vi "Motor_Plus_Impedance_controller_using_force_feedback_only.vi"() -> ()   [LabVIEW 2016]
uses:
  <vilib>/Platform/TimedLoop/XDataNode/timing_clust.ctl
  <vilib>/Platform/TimedLoop/XDataNode/nitl_modes.ctl
  <vilib>/Platform/TimedLoop/XDataNode/wakeup.ctl
  <vilib>/Platform/TimedLoop/XDataNode/loadnilvce.vi
  <vilib>/Motion/Express/_s/nimc.fb.resetPosition.resetPosition.axis.vi
  <vilib>/Motion/Express/_s/nimc.fb.read.readFaults.axis.vi
  <vilib>/Motion/Express/_s/nimc.fb.read.readExecutionStatus.axis.vi
  <vilib>/Motion/Express/_s/nimc.fb.straightLineMove.startStraightLineMove.axis.modeRelative.0.vi
  <vilib>/Motion/Express/_s/nimc.fb.read.readExecutionData.axis.vi
  <vilib>/Motion/Express/_s/nimc.fb.straightLineMove.startStraightLineMove.axis.modeAbsolute.0.vi
  <vilib>/Motion/Express/_s/nimc.ax.power.power.axis.vi
  <vilib>/Motion/Express/_s/nimc.fb.stopMove.stop.axis.modeDecelerate.vi
  <vilib>/Motion/Express/_s/nimc.ex.power.power.axis.vi
  <vilib>/Platform/TimedLoop/XDataNode/XDataNode.xnode
  <vilib>/Motion/BlockNode/FB.NIMotion.xnode
  <vilib>/functionblocks/FB Property/FB Overlay DBL.ctl
  <vilib>/Platform/TimedLoop/XDataNode/XDNodeRunTimeDep.lvlib
panel:
  in  "Tab Control":enum32{"Record", "PID Check", "Load Cell Check"}(tab)
  out "Crank Position, rev":dbl(knob) scale=-100.0..100.0
  out "Crank Speed, rev/s":dbl(knob) scale=0.0..300.0
  out "Motor Torque, Nm":dbl(knob) scale=-5.0..5.0
  out "Load Cell Force, N":dbl(knob) scale=-50.0..50.0
  out "Recording?":bool
  in  "Record Data?":bool
  in  "Path":path=path "C:/ni-rt/LabVIEW Data/Ashley Carter"
  in  "File Name:":string="2015_03_31_60rpm_20rev_B_1.tdms"
  in  "Prime New File?":bool
  out "File being written to:":path
  out "FIFO Timer, Sec":dbl
  out "FIFO motor position, rev":dbl
  out "FIFO motor velocity, rev/s":dbl
  out "FIFO motor torque, Nm":dbl
  out "FIFO Load cell, V":dbl
  out "FIFO File logging trigger":dbl
  out "# FIFO elements remaining in buffer":u32
  out "Data File Crank Angle Sample Resolution, degrees of crank rotation":dbl
  out "Motor Control PID Check":cluster{dbl, dbl}(graph)
  out "Load Cell Check":cluster{dbl, dbl, dbl}(graph)
  out "Logging loop duration, ms":u32
  out "Control loop duration, ms":u32
  out "RPM LIMITING!":bool
  in  "desired motor\nposition":dbl
  in  "Move to Position?":bool
  in  "Reset Position?":bool
  out "fault occurred":bool
  out "System reported fault codes":i32[](array[numeric])
  out "Load cell, V":dbl format="%.3f"
  out "motor torque, Nm":dbl format="%.3f"
  out "motor velocity, rev/s":dbl format="%.3f"
  out "motor position, rev":dbl format="%.3f"
  out "Timer, sec":dbl format="%.3f"
  out "drive enabled":bool
  out "axis enabled":bool
  out "move complete":bool
  in  "STOP VI":bool
  in  "Enable Axis Control":bool
  in  "Enable Motor Drive":bool
  in  "crank rpm":dbl=60.0
  in  "crank no. revolutions":dbl=5.0
  in  "EMERGENCY MOTOR STOP":bool
  in  "Start Test?":bool
  # "Impedance Motor Controller"
  # "Impedance Control Basic Data Recording and PID Tuning"
  # "(This only stops the move, the drive remains enabled!!!)"
  # "Crank RPM and no. Revolutions"
  # "Raw Data from System"
  # "Suggested process to align above reported motor position to test rig TDC:\n\nWith the Enable Motor Drive and Enable Axis Control switches set to off\nmanually rotate the 'engine' to BDC then click Enable Motor Control and \nEnable Axis Control. 'motor position, rev' above then reports a value. Press the\nbutton 'Reset Position'. The motor encoder reported position is now zeroed to\nBDC. In the 'Desired Motor Position' box set a value of 1 and press the button\n'Move to Position?'. The 'engine' should move to approx. TDC. Then press\n'Reset Position' again to zero at TDC. Fine adjustment of TDC can be achieved\nby putting small corrections into 'desired motor position' and pressing 'move to\nposition?' followed by 'Reset Position. \n\nAfter each run, Reset Position can be pressed to set the motor position back to \nzero for the next run to make calculation of piston position in post data analysis\neasier."
  # "Note: to record to a new file, run this\nprogram then type the FILE NAME and\nthen pres Prime New File - this then \ncreates and opens the file ready to record\ndata to the file.\n\nThen press 'Record Data'; data will be \nrecorded when the 'Start Test' button is \npressed"
  # "Note: the control loop time interval is 5ms (200Hz), data is scanned at this same\nfrequency irrespective of crank rpm set.\n\nThus, the data sample resolution in Crank Angle Degrees  can be calculated as:\n\n((rpm/60) x 360))/200Hz = 0.03 x crank rpm\n\nso at 100 rpm the sample resolution is 3 crank angle degrees"
  # "To tune the PID control, go to the project and right-click on Axis 1 and select Properties.\nThen click the 'Position Loop' icon. Edit the kp, ki and kd as required. \nDefault twin crank rig values: kp=50, ki=0, kd=1000"
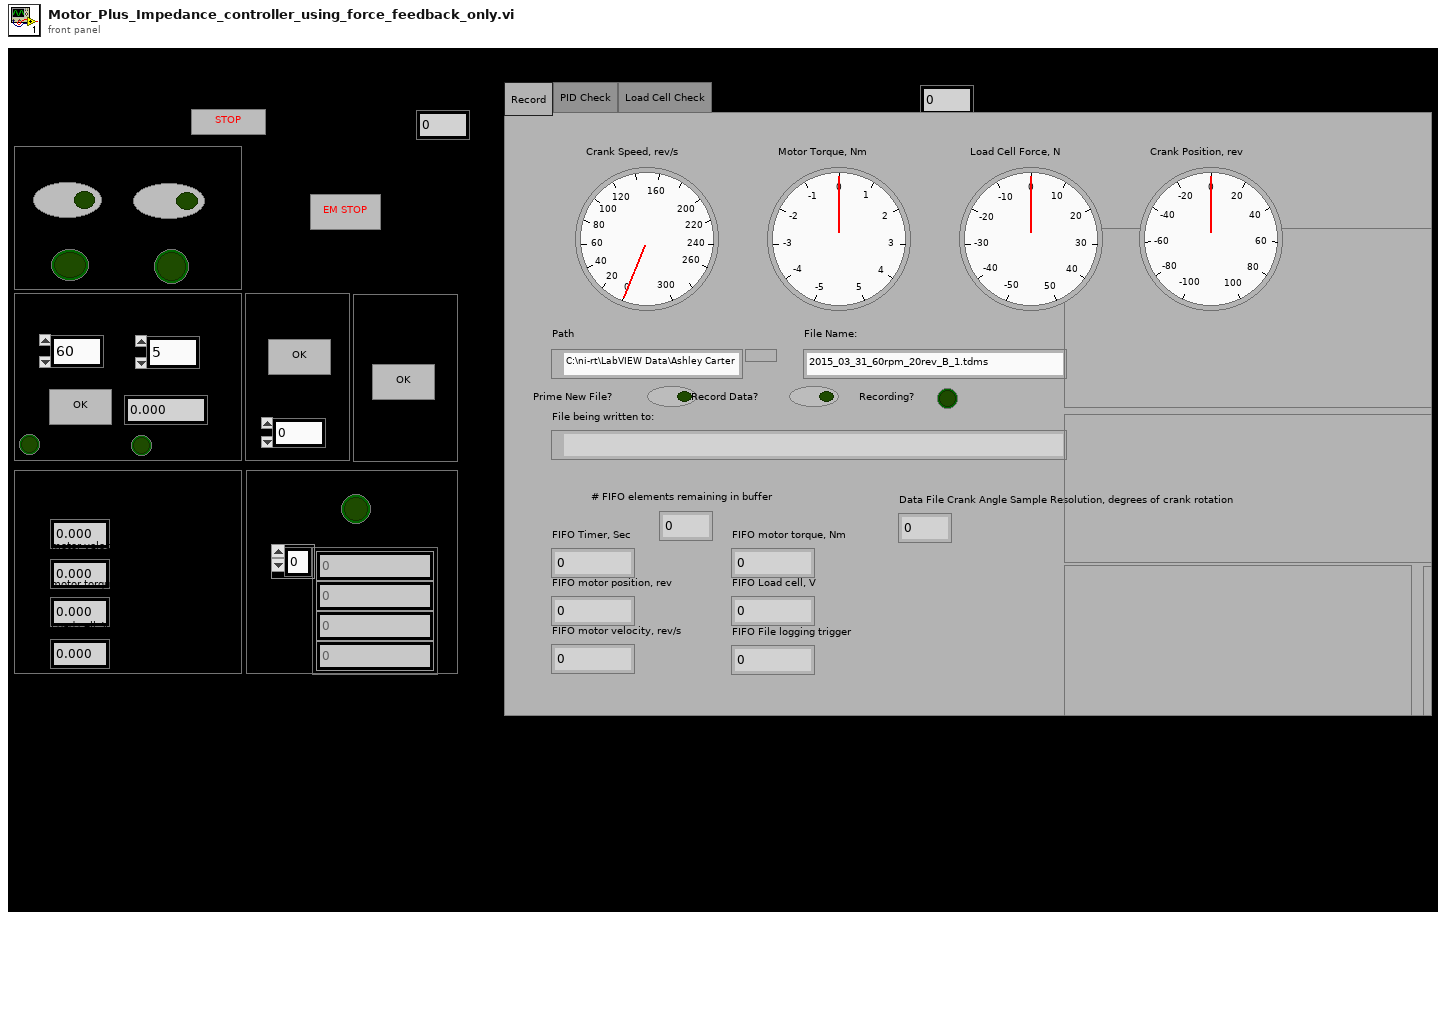
[diagram p1: front panel]
types:
  T1 = enum16{"big-endian, network order", "native, host order", "little-endian"}
  T2 = enum16{"open", "open or create", "create or replace", "create", "open (read-only)"}
  T3 = typedef "XDNodeRunTimeDep.lvlib/timing_clust.ctl" = cluster{"Expected End [f-1]":u64, "Actual End [f-1]":u64, "Finished Late? [f-1]":bool, "Expected End [i-1]":u64, "Actual End [i-1]":u64, "Finished Late? [i-1]":bool, "Expected Start [i]":u64, "Actual Start [i]":u64, "Expected Start [f]":u64, "Actual Start [f]":u64, "Source Name":string, "Structure Name":string, "Period":i64, "Deadline":i64, "Offset":i64, "Start":i64, "Priority":i32, "Timeout":i32, "Mode":T4, "Wakeup Reason":T5, "Error":errorcluster, "Source Type":string, "Secondary Source Type":string, "Global End Time":u64, "Global Start Time":u64, "Frame Duration":u64, "Iteration Duration":u64, "Assigned CPU":i32, "I/O Scan Engine Mode":u32}
  T4 = typedef "XDNodeRunTimeDep.lvlib/nitl_modes.ctl" = enum32{"No Change", "Process missed periods, maintain original phase", "Discard missed periods, maintain original phase", "Process missed periods, ignore original phase", "Discard missed periods, ignore original phase"}
  T5 = typedef "XDNodeRunTimeDep.lvlib/wakeup.ctl" = enum32{"Normal", "Aborted", "Asynchronous wakeup", "Timing source error", "Timed loop error", "Timeout"}
  T6 = cluster{dbl, "position":dbl, "velocity":dbl, "torque":dbl, "Double":dbl, i16, "STOP VI":bool}
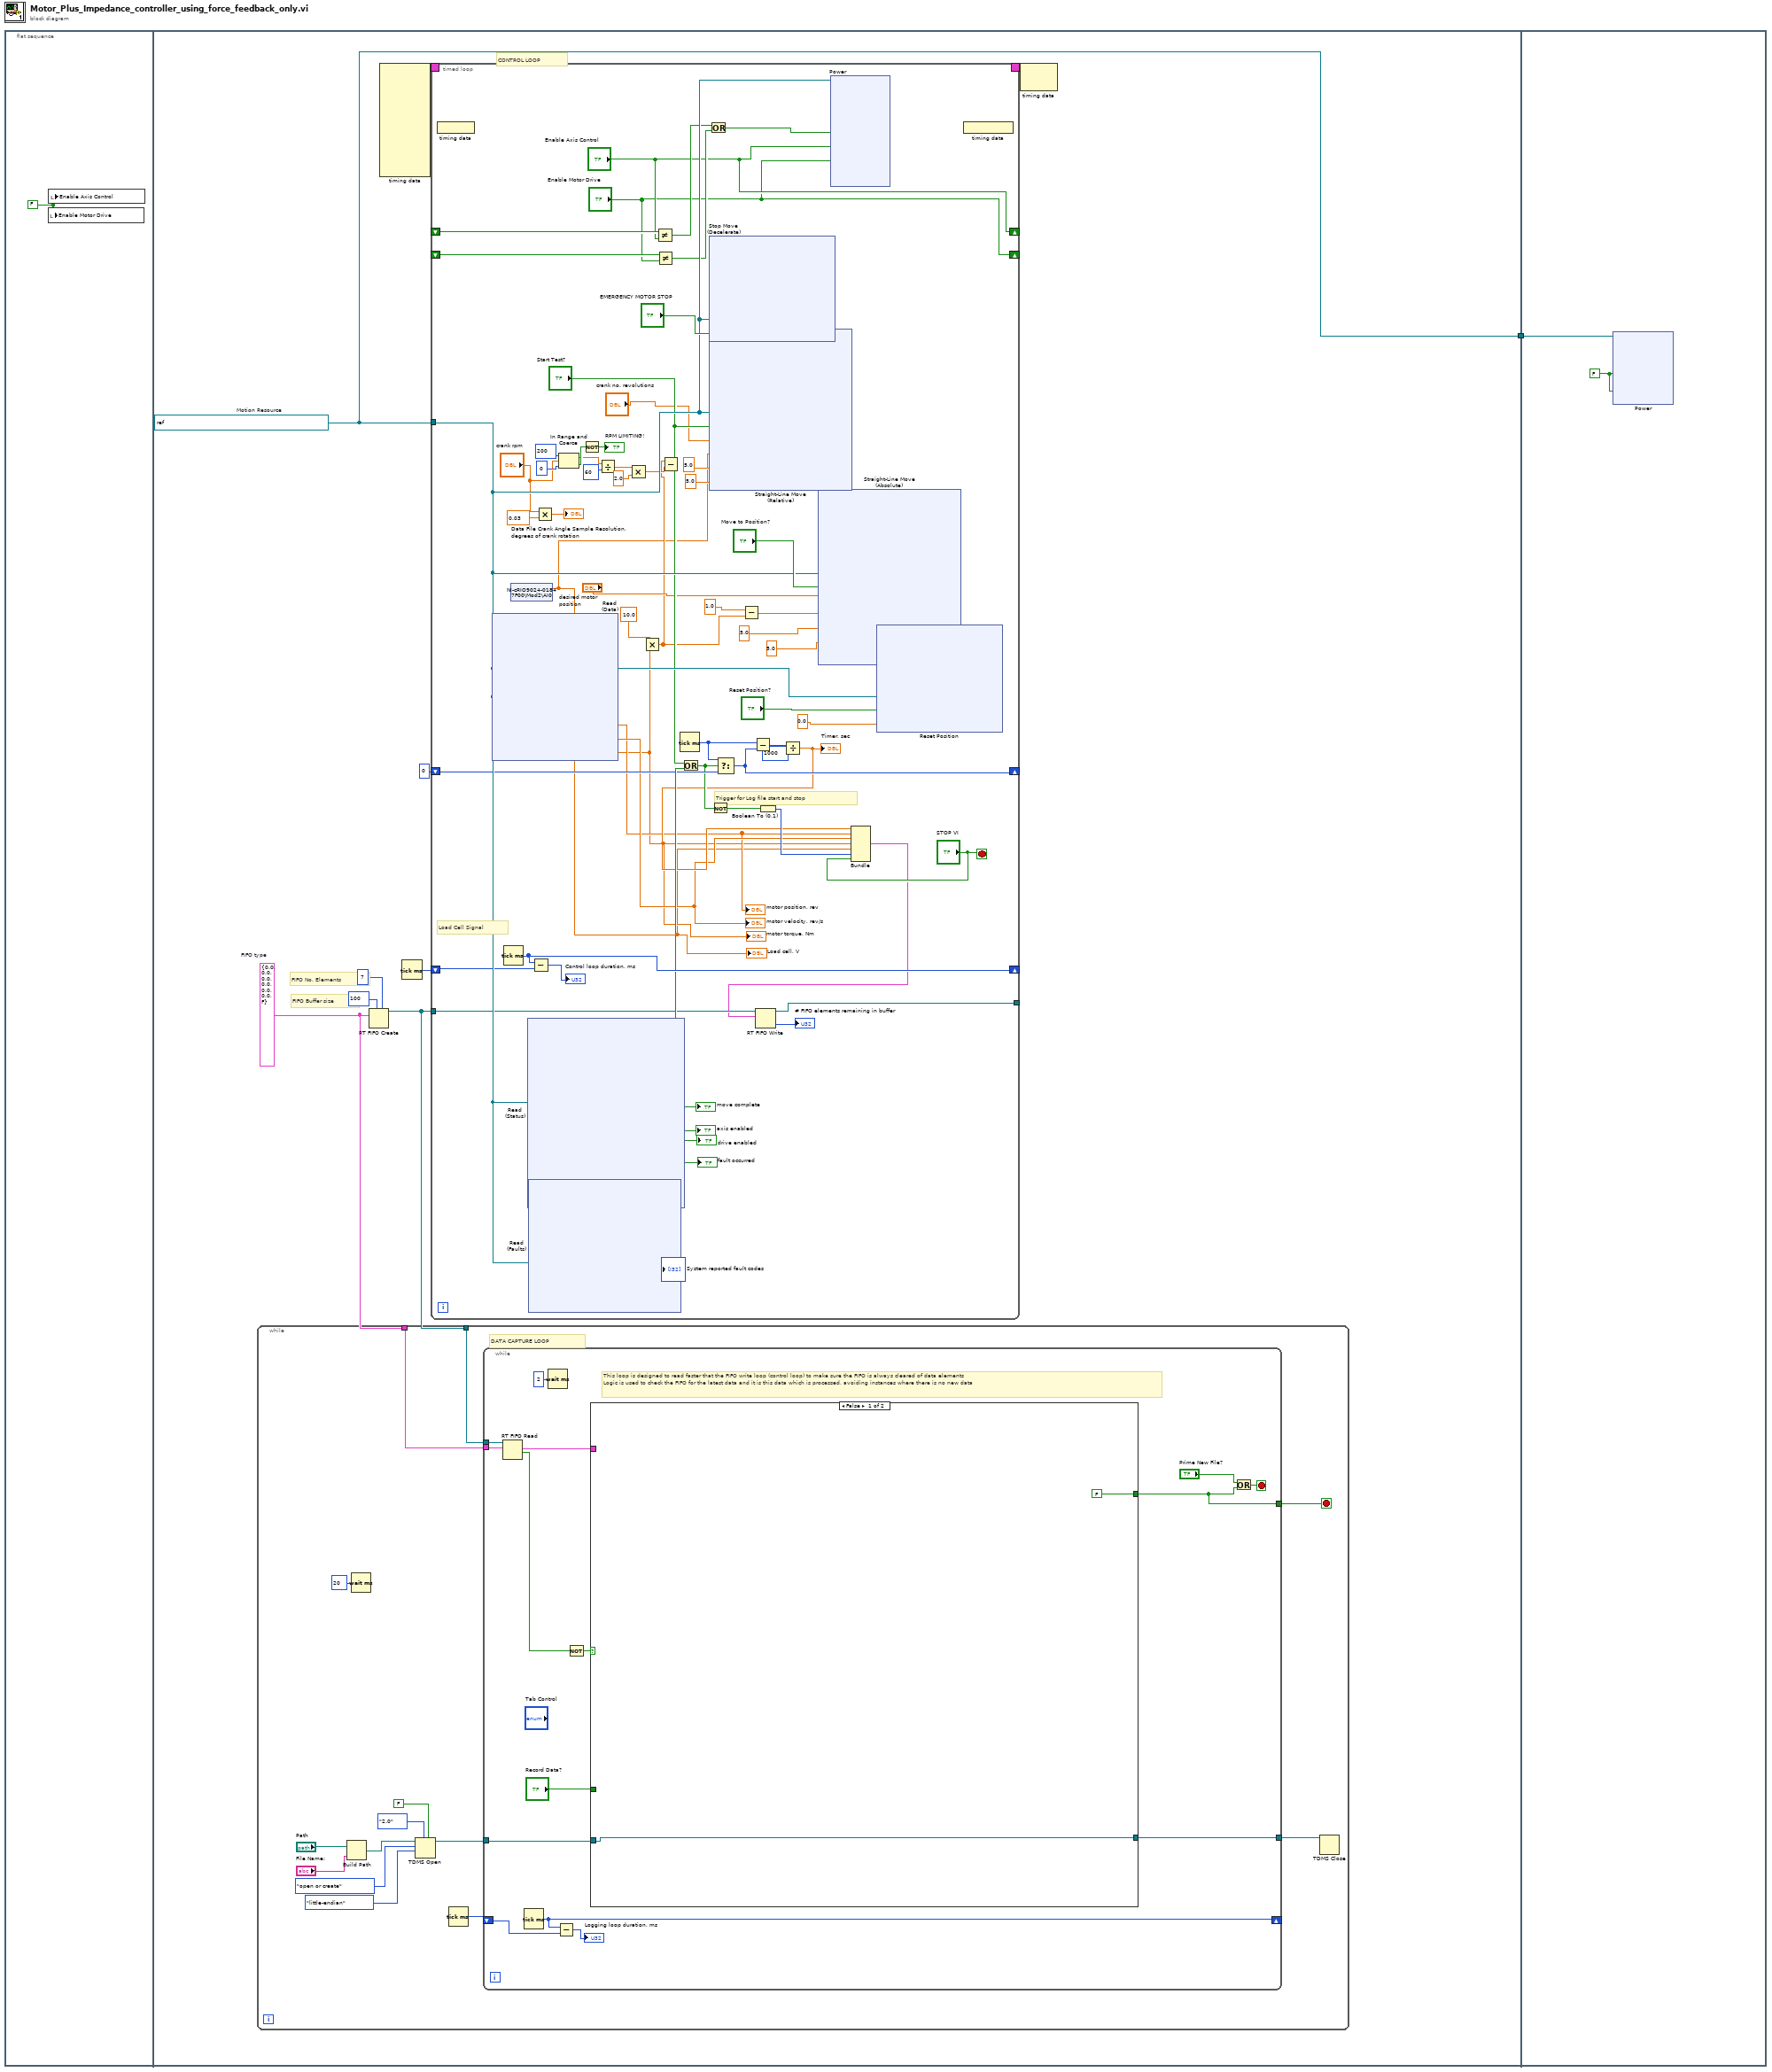
[diagram p0: block diagram]
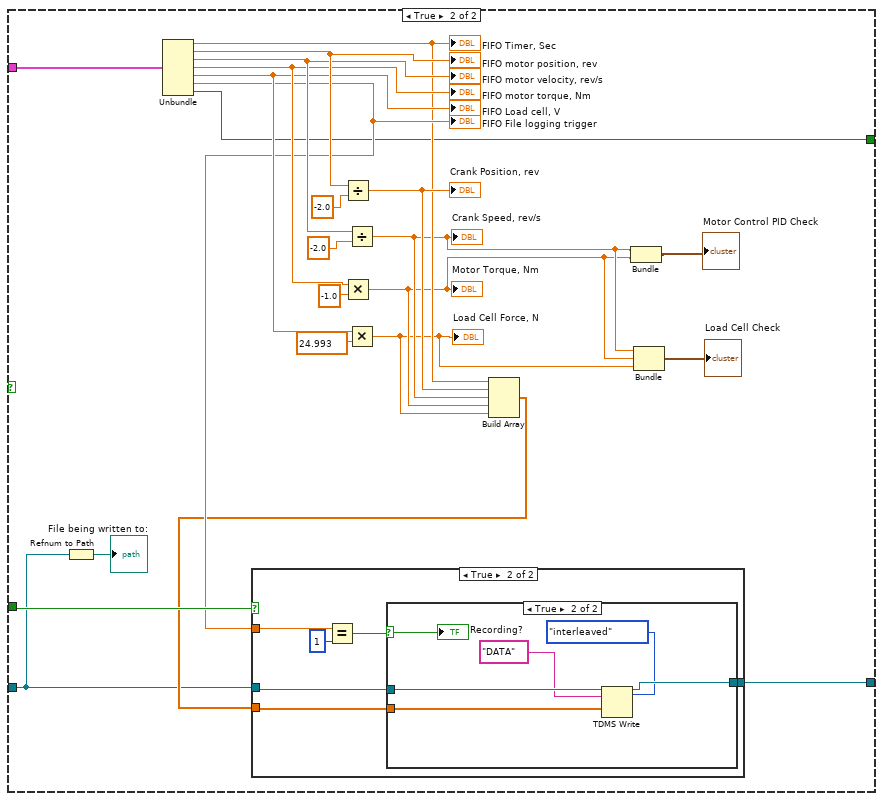
[diagram p2: hidden frame]
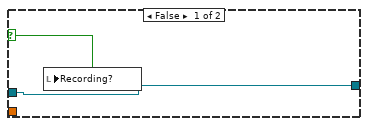
[diagram p4: hidden frame]
diagram:
  n1 = flat-sequence {
    tunnel: [w11] -> w1
    tunnel: w1 -> [w274]
    frame #0 {
      w2 = FALSE
      n2 = local write "Enable Motor Drive"(w2) -> ()
      n3 = local write "Enable Axis Control"(w2) -> ()
    }
    frame #1 {
      w4 = cluster{dbl, dbl, dbl, dbl, dbl, dbl, bool} {0.0, 0.0, 0.0, 0.0, 0.0, 0.0, FALSE}  # FIFO type
      w11 = refnum<k21> "nism://NI-cRIO9024-01847F00/Axis 1"  # Motion Resource
      # "FIFO No. Elements"
      # "FIFO Buffer size"
      # "CONTROL LOOP"
      n4 = RT FIFO Create(1:w4, 4:u32 100 ("size (10)"), 6:u32 7 ("elements in array (1)")) -> (8:w5:refnum<k33>)  [unwired: 5 in, 2 out]
      n5 = while {
        tunnel: w5 -> [w25]
        tunnel: w4 -> [w24]
        stop <- w13 stop-if-true
        # "DATA CAPTURE LOOP"
        n6 = Build Path(base path="Path", name or relative path="File Name:") -> (appended path=w18:path)
        n7 = Wait (ms)(milliseconds to wait=20) -> ()  [unwired: 1 out]
        n8 = TDMS Open(5:FALSE ("create index file? (T)"), 7:enum16{"1.0", "2.0"}."2.0" ("file format version (2.0)"), 9:T1."little-endian" ("byte order (2:little-endian)"), 10:T2."open or create" ("operation (0:open)"), 11:w18) -> (3:w15:refnum<k34>)  [unwired: 2 in, 1 out]
        n9 = Tick Count (ms)() -> (millisecond timer value=w23:u32)
        n10 = while {
          tunnel: w25 -> [w40]
          tunnel: w24 -> [w39]
          shift-right: [w35] -> _
          shift-left: w23 -> [w36]
          tunnel: w15 -> [w33]
          tunnel: [w32] -> w14
          tunnel: [w29] -> w13
          stop <- w31 stop-if-true
          # "This loop is designed to read faster that the FIFO write loop (control loop) to make sure the FIFO is always cleared of data elements\nLogic is used to check the FIFO for the latest data and it is this data which is processed, avoiding instances where there is no new data"
          n11 = RT FIFO Read(0:w40, 1:w39) -> (9:w38:cluster{dbl, dbl, dbl, dbl, dbl, dbl, bool}, 10:w27:bool)  [unwired: 2 in, 3 out]
          n12 = Tick Count (ms)() -> (millisecond timer value=w35:u32)
          n13 = Wait (ms)(milliseconds to wait=2) -> ()  [unwired: 1 out]
          n14 = Subtract(x=w35, y=w36) -> (x-y=→"Logging loop duration, ms":u32)
          n15 = Not(x=w27) -> (.not. x?=w28:bool)
          n16 = case shown="False" w28 {
            tunnel: w38 -> [_ w65]
            tunnel: "Record Data?" -> [_ w64]
            tunnel: w33 -> [w41 w49]
            tunnel: [w41 w54] -> w32
            tunnel: [FALSE w50] -> w29
            frame False {
            }
            frame True {
              n17 = Refnum to Path(1:w49) -> (0:→"File being written to:":path)
              n18 = Unbundle(w65) -> (w52:dbl, w62:dbl, w60:dbl, w58:dbl, w56:dbl, w55:dbl, w50:bool)
              "FIFO Timer, Sec" <- w52
              "FIFO motor position, rev" <- w62
              "FIFO motor velocity, rev/s" <- w60
              "FIFO motor torque, Nm" <- w58
              "FIFO Load cell, V" <- w56
              "FIFO File logging trigger" <- w55
              n19 = Divide(x=w62, y=-2.0) -> (x/y=w53:dbl)
              "Crank Position, rev" <- w53
              n20 = Multiply(x=w58, y=-1.0) -> (x*y=w44:dbl)
              "Motor Torque, Nm" <- w44
              n21 = Divide(x=w60, y=-2.0) -> (x/y=w45:dbl)
              "Crank Speed, rev/s" <- w45
              n22 = Multiply(x=w56, y=24.993) -> (x*y=w43:dbl)
              "Load Cell Force, N" <- w43
              n23 = Build Array(w52, w53, w45, w44, w43) -> (w51:dbl[])
              n24 = case shown="True" w64 {
                tunnel: w51 -> [_ w72]
                tunnel: w55 -> [_ w69]
                tunnel: w49 -> [w66 w68]
                tunnel: [w66 w67] -> w54
                frame False {
                }
                frame True {
                  n25 = Equal?(x=w69, y=1) -> (x = y?=w71:bool)
                  n26 = case shown="True" w71 {
                    selector: w71 -> [w74 w80]
                    tunnel: w72 -> [_ w75]
                    tunnel: w68 -> [w73 w79]
                    tunnel: [w73 w77] -> w67
                    frame False {
                      n27 = local write "Recording?"(w74) -> ()
                    }
                    frame True {
                      n28 = TDMS Write(0:w79, 1:enum16{"decimated", "interleaved"}."interleaved" ("data layout (0:decimated)"), 5:"DATA" ("group name in (Untitled)"), 9:w75) -> (4:w77:refnum<k34>)  [unwired: 2 in, 3 out]
                      "Recording?" <- w80
                    }
                  }
                }
              }
              n29 = Bundle(w45, w44) -> (→"Motor Control PID Check":cluster{dbl, dbl})  [unwired: 1 in]
              n30 = Bundle(w45, w44, w43) -> (→"Load Cell Check":cluster{dbl, dbl, dbl})  [unwired: 1 in]
            }
          }
          n31 = Or(x="Prime New File?", y=w29) -> (x .or. y?=w31:bool)
        }
        n32 = TDMS Close(11:w14) -> ()  [unwired: 1 in, 2 out]
      }
      n33 = node-c288() -> (w10:T3)  [unwired: 10 in]
      n34 = Tick Count (ms)() -> (millisecond timer value=w8:u32)
      n35 = timed-loop {
        tunnel: w11 -> [w128]
        timing: w10 -> [_]
        timing-out: [_] -> w9
        shift-right: [w122] -> _
        shift-left: w8 -> [w123]
        shift-right: ["Enable Axis Control"] -> _
        shift-left: _ -> [w117]
        shift-right: ["Enable Motor Drive"] -> _
        shift-left: _ -> [w116]
        tunnel: w5 -> [w107]
        tunnel: [w106] -> _
        shift-right: [w99] -> _
        shift-left: 0 -> [w101]
        stop <- "STOP VI" stop-if-true
        # "Trigger for Log file start and stop"
        # "Load Cell Signal"
        n36 = node-c288() -> ()  [unwired: 1 in]
        n37 = xnode "Read\n(Data)"("resource"=w128) -> ("position"=w89:dbl, "velocity"=w90:dbl, "torque"=w83:dbl)  [unwired: 1 in, 3 out]
        "motor position, rev" <- w89
        "motor velocity, rev/s" <- w90
        "motor torque, Nm" <- w83
        n38 = Tick Count (ms)() -> (millisecond timer value=w122:u32)
        n39 = shared-variable "NI-cRIO9024-01847F00\\Mod2\\AI0"() -> (w81:dbl)  [unwired: 1 in, 1 out]
        "Load cell, V" <- w81
        n40 = xnode "Read\n(Status)"("resource"=w128) -> ("move complete"=w108:bool, "axis enabled"=→"axis enabled":bool, "drive enabled"=→"drive enabled":bool, "fault occurred"=→"fault occurred":bool)  [unwired: 1 in, 5 out]
        "move complete" <- w108
        n41 = xnode "Read\n(Faults)"("resource"=w128) -> ("fault code[] out"=→"System reported fault codes":i32[])  [unwired: 2 in, 4 out]
        n42 = Subtract(x=w122, y=w123) -> (x-y=→"Control loop duration, ms":u32)
        n43 = Multiply(x="crank rpm", y=0.03) -> (x*y=→"Data File Crank Angle Sample Resolution, degrees of crank rotation":dbl)
        n44 = In Range and Coerce(upper limit=200, x="crank rpm", lower limit=0) -> (coerced(x)=w119:dbl, In Range?=w124:bool)
        n45 = Not(x=w124) -> (.not. x?=→"RPM LIMITING!":bool)
        n46 = Divide(x=w119, y=60) -> (x/y=w120:dbl)
        n47 = Multiply(x=w120, y=2.0) -> (x*y=w86:dbl)
        n48 = Multiply(x=10.0, y=w83) -> (x*y=w82:dbl)
        n49 = Not Equal?(x=w117, y="Enable Axis Control") -> (x != y?=w115:bool)
        n50 = Not Equal?(x=w116, y="Enable Motor Drive") -> (x != y?=w114:bool)
        n51 = Subtract(x=w82, y=w86) -> ()  [unwired: 1 out]
        n52 = Tick Count (ms)() -> (millisecond timer value=w100:u32)
        n53 = Or(x="Start Test?", y=w108) -> (x .or. y?=w98:bool)
        n54 = Or(x=w115, y=w114) -> (x .or. y?=w113:bool)
        n55 = xnode "Stop Move\n(Decelerate)"("resource"=w128, "execute"="EMERGENCY MOTOR STOP") -> ()  [unwired: 1 in, 3 out]
        n56 = xnode "Straight-Line Move\n(Relative)"("resource"=w128, "execute"="Start Test?", "position"="crank no. revolutions", "velocity"=w81, "acceleration"=5.0, "deceleration"=5.0) -> ()  [unwired: 1 in, 3 out]
        n57 = Not(x=w98) -> (.not. x?=w110:bool)
        n58 = Select(t=w100, s=w98, f=w101) -> (s? t:f=w99:u32)
        n59 = Subtract(x=1.0, y=w82) -> (x-y=w85:dbl)
        n60 = Subtract(x=w100, y=w99) -> (x-y=w97:u32)
        n61 = Boolean To (0,1)(Boolean=w110) -> (0, 1=w105:i16)
        n62 = Divide(x=w97, y=1000) -> (x/y=w95:dbl)
        "Timer, sec" <- w95
        n63 = xnode "Straight-Line Move\n(Absolute)"("resource"=w128, "execute"="Move to Position?", "position"="desired motor\nposition", "velocity"=w85, "acceleration"=5.0, "deceleration"=5.0) -> ()  [unwired: 1 in, 3 out]
        n64 = xnode ("Power")("execute"=w113, "enable axis"="Enable Axis Control", "enable drive"="Enable Motor Drive", "resource"=w128) -> ()  [unwired: 1 in, 6 out]
        n65 = Bundle(w95, "position"=w89, "velocity"=w90, "torque"=w83, "Double"=w81, w105, "STOP VI"="STOP VI") -> (w103:T6)  [unwired: 1 in]
        n66 = RT FIFO Write(0:w107, 1:w103) -> (7:→"# FIFO elements remaining in buffer":u32, 8:w106:refnum<k33>)  [unwired: 3 in, 2 out]
        n67 = xnode "Reset Position"("resource"=w128, "execute"="Reset Position?", "position"=0.0) -> ()  [unwired: 1 in, 3 out]
        n68 = node-c288() -> ()  [unwired: 1 out]
      }
      n69 = node-c288(w9) -> ()  [unwired: 1 out]
    }
    frame #2 {
      w275 = FALSE
      n70 = xnode ("Power")("enable axis"=w275, "enable drive"=w275, "resource"=w274) -> ()  [unwired: 1 in, 2 out]
    }
  }
